vi "Read Valid Relation.vi"(11 "Base Teller in":refnum<class "Base Teller.lvclass">) -> (2 "Valid Relation":bool)   [LabVIEW 2020, in "jettl.lvlib" / "Base Teller.lvlib" / "Base Teller.lvclass"]
uses:
  Base Teller.lvclass
  Base Teller.lvclass/Base Teller.ctl
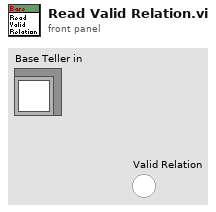
[diagram p1: front panel]
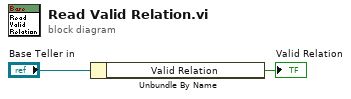
[diagram p0: block diagram]
diagram:
  n1 = Unbundle By Name("Base Teller in") -> ("Valid Relation"=→"Valid Relation":bool)
